vi "Set First Tab to Node Text.vi"(8 "error in (no error)":errorcluster, 11 "Target in":refnum<class "Target.lvclass">) -> (0 "error out":errorcluster)   [LabVIEW 2015, in "Configuration Tool.lvlib"]
uses:
  Configuration Tool.lvlib
  Classes/Target/Target.lvclass
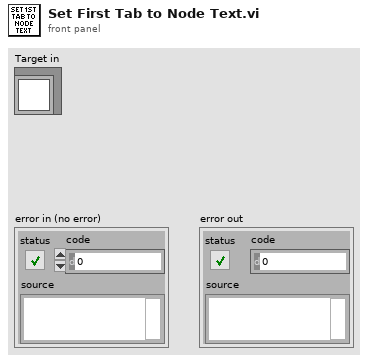
[diagram p1: front panel]
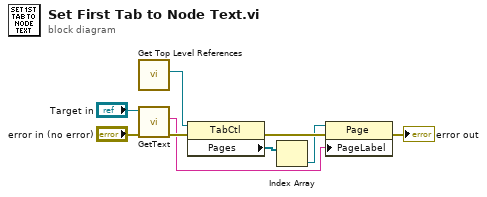
[diagram p0: block diagram]
diagram:
  n1 = call "Get Top Level References.vi"() -> ("Main UI Tab Ref"=w1:refnum<vi>)  [unwired: 9 in, 2 out]
  n2 = call-dynamic "GetText.vi"("error in"="error in (no error)", "node in"="Target in") -> ("error out"=w6:errorcluster, "text"=w4:string)  [unwired: 5 in, 3 out]
  n3 = property on="Property Node" class="TabCtl"(reference=w1, error in=w6) -> (error out=w7:errorcluster, "Pages"=w3:refnum<vi>[])  [unwired: 1 out]
  n4 = Index Array(array=w3) -> (element=w2:refnum<vi>)  [unwired: 1 in]
  n5 = property class="Page"(reference=w2, error in=w7, "PageLabel"=w4) -> (error out=→"error out":errorcluster)  [unwired: 1 out]
